vi "GetAllPaths.vi"() -> (1 "Server Folder":path, 2 "BlankServer":path, 3 "Console Path":path)   [LabVIEW 2013]
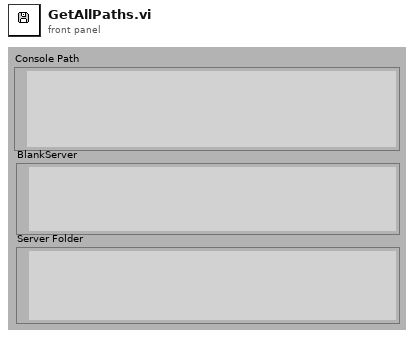
[diagram p1: front panel]
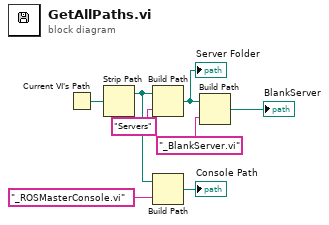
[diagram p0: block diagram]
diagram:
  n1 = Current VI's Path() -> (path=w8:path)
  n2 = Strip Path(path=w8) -> (stripped path=w3:path)  [unwired: 1 out]
  n3 = Build Path(base path=w3, name or relative path="Servers") -> (appended path=w1:path)
  "Server Folder" <- w1
  n4 = Build Path(base path=w3, name or relative path="_ROSMasterConsole.vi") -> (appended path=→"Console Path":path)
  n5 = Build Path(base path=w1, name or relative path="_BlankServer.vi") -> (appended path=→"BlankServer":path)
